vi "qp_fill data.vi"(7 "x0":dbl[](array[numeric]), 8 "inequality constraints":cluster{"D":dbl[][], "Imin":dbl[], "Imax":dbl[]}, 9 "equality constraints":cluster{"A":dbl[][], "b":dbl[]}, 10 "parameter bounds":cluster{"Xmin":dbl[], "Xmax":dbl[]}, 11 "objective function":cluster{"Q":dbl[][], "c":dbl[]}) -> (3 "qp data in":T1)   [LabVIEW 2018, in "NI_Gmath.lvlib"]
uses:
  NI_Gmath.lvlib
  qp_problem data.ctl
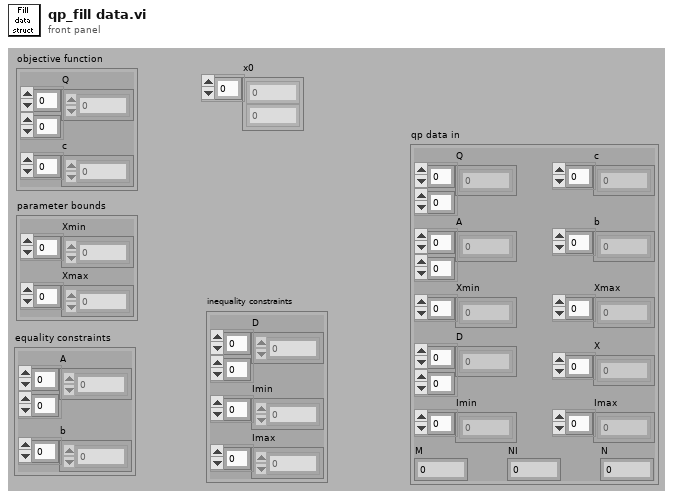
[diagram p1: front panel]
types:
  T1 = typedef "NI_Gmath.lvlib/qp_problem data.ctl" = cluster{"Q":dbl[][], "c":dbl[], "A":dbl[][], "b":dbl[], "Xmin":dbl[], "Xmax":dbl[], "M":i32, "N":i32, "D":dbl[][], "Imax":dbl[], "Imin":dbl[], "NI":i32, "X":dbl[]}
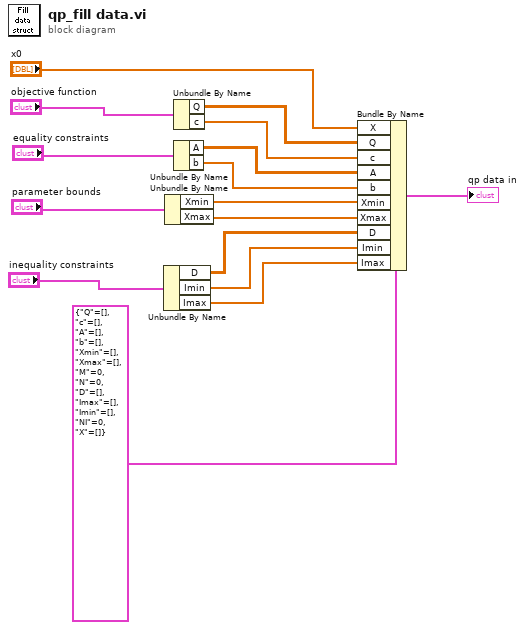
[diagram p0: block diagram]
diagram:
  n1 = Unbundle By Name("inequality constraints") -> ("D"=w4:dbl[][], "Imin"=w3:dbl[], "Imax"=w2:dbl[])
  n2 = Unbundle By Name("parameter bounds") -> ("Xmin"=w6:dbl[], "Xmax"=w5:dbl[])
  n3 = Unbundle By Name("objective function") -> ("Q"=w10:dbl[][], "c"=w9:dbl[])
  n4 = Unbundle By Name("equality constraints") -> ("A"=w8:dbl[][], "b"=w7:dbl[])
  n5 = Bundle By Name(cluster=T1 {"Q"=[], "c"=[], "A"=[], "b"=[], "Xmin"=[], "Xmax"=[], "M"=0, "N"=0, "D"=[], "Imax"=[], "Imin"=[], "NI"=0, "X"=[]} ("qp data in"), "X"="x0", "Q"=w10, "c"=w9, "A"=w8, "b"=w7, "Xmin"=w6, "Xmax"=w5, "D"=w4, "Imin"=w3, "Imax"=w2) -> (→"qp data in":T1)
